vi "to_be_2_string.vi"(11 "string 2":string) -> (3 "substring 2":string)   [LabVIEW 2017]
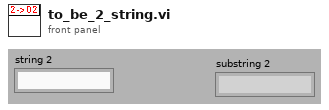
[diagram p1: front panel]
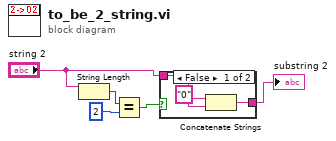
[diagram p0: block diagram]
diagram:
  n1 = String Length(string="string 2") -> (length=w5:i32)
  n2 = Equal?(x=w5, y=2) -> (x = y?=w3:bool)
  n3 = case shown="False" w3 {
    tunnel: "string 2" -> [w8 w9]
    tunnel: [w6 w9] -> w1
    frame False {
      n4 = Concatenate Strings("0" ("string"), w8) -> (w6:string)
    }
    frame True {
    }
  }
  "substring 2" <- w1
